vi "nirvififoUniquifyingName.vi"(7 "parent VI":refnum<vi>, 12 "local?":bool) -> (8 "uniquifier":string)   [LabVIEW 2020]
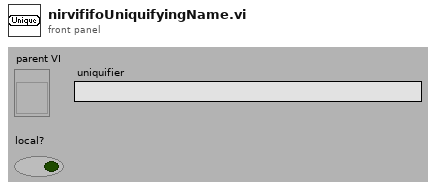
[diagram p1: front panel]
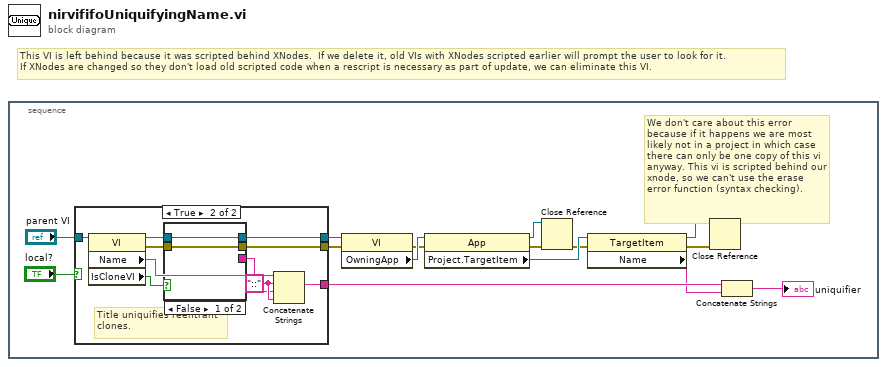
[diagram p0: block diagram]
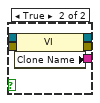
[diagram p3: hidden frame]
diagram:
  # "This VI is left behind because it was scripted behind XNodes.  If we delete it, old VIs with XNodes scripted earlier will prompt the user to look for it.\nIf XNodes are changed so they don't load old scripted code when a rescript is necessary as part of update, we can eliminate this VI."
  n1 = stacked-sequence {
    frame #0 {
      # "We don't care about this error because if it happens we are most likely not in a project in which case there can only be one copy of this vi anyway. This vi is scripted behind our xnode, so we can't use the erase error function (syntax checking)."
      n2 = case shown="True" "local?" {
        tunnel: [_ w21] -> w8
        tunnel: [_ w25] -> w5
        tunnel: "parent VI" -> [w16 w24]
        tunnel: [w16 w19] -> w2
        frame False {
        }
        frame True {
          w23 = "::" ("string")
          # "Title uniquifies reentrant\nclones."
          n3 = property class="VI"(reference=w24) -> (reference out=w20:refnum<vi>, error out=w18:errorcluster, "Name"=w26:string, "IsCloneVI"=w22:bool)  [unwired: 1 in]
          n4 = case shown="False" w22 {
            tunnel: [w28 w30] -> w21
            tunnel: w20 -> [w27 w32]
            tunnel: [w27 w31] -> w19
            tunnel: w18 -> [w28 w33]
            tunnel: [_ w29] -> w17
            frame False {
            }
            frame True {
              n5 = property class="VI"(reference=w32, error in=w33) -> (reference out=w31:refnum<vi>, error out=w30:errorcluster, "Clone Name"=w29:string)
            }
          }
          n6 = Concatenate Strings(w26, w23, w17, w23) -> (w25:string)
        }
      }
      n7 = property class="VI"(reference=w2, error in=w8) -> (error out=w1:errorcluster, "OwningApp"=w14:refnum<vi>)  [unwired: 1 out]
      n8 = property class="App"(reference=w14, error in=w1) -> (reference out=w12:refnum<vi>, error out=w13:errorcluster, "Project.TargetItem"=w11:refnum<vi>)
      n9 = Close Reference(reference=w12, error in (no error)=w13) -> (error out=w9:errorcluster)
      n10 = property class="TargetItem"(reference=w11, error in=w9) -> (reference out=w15:refnum<vi>, error out=w10:errorcluster, "Name"=w4:string)
      n11 = Close Reference(reference=w15, error in (no error)=w10) -> ()  [unwired: 1 out]
      n12 = Concatenate Strings(w5, w4) -> (→"uniquifier":string)
    }
  }
